vi "Not A Refnum.vi"(8 "error in (no error)":errorcluster, 11 "Log File in":refnum<class "Log File.lvclass">) -> (0 "error out":errorcluster, 2 "Not a Refnum?":bool, 3 "Log File out":refnum<class "Log File.lvclass">)   [LabVIEW 2015, in "Log File.lvclass"]
uses:
  Log File.lvclass
  Log File.lvclass/Log File.ctl
  TDMS Log File/TDMS Log File.lvclass
  Text Log File/Text Log File.lvclass
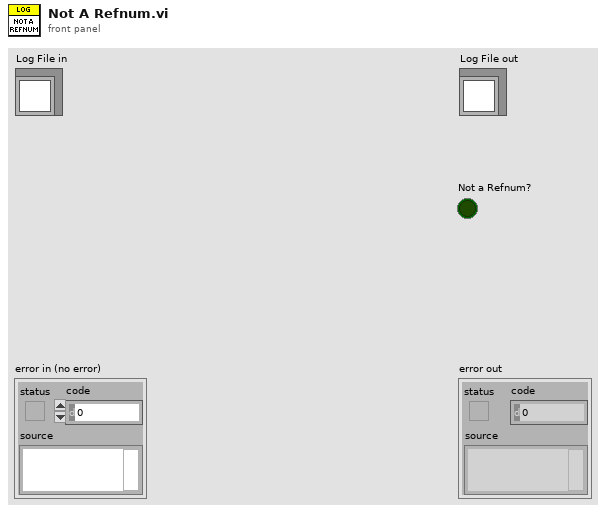
[diagram p1: front panel]
types:
  T1 = typedef "Log File.lvclass/Log File Type.ctl" = enum16{"Default", "TDMS", "Text"}
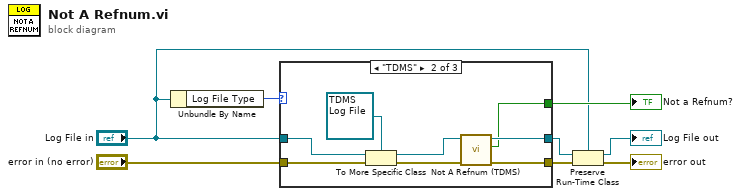
[diagram p0: block diagram]
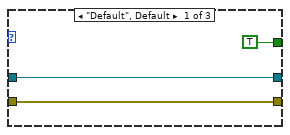
[diagram p2: hidden frame]
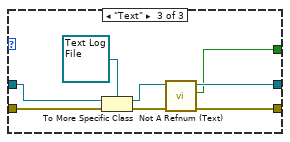
[diagram p3: hidden frame]
diagram:
  n1 = Unbundle By Name("Log File in") -> ("Log File Type"=w8:T1)
  n2 = case shown="\"TDMS\"" w8 {
    tunnel: "error in (no error)" -> [w11 w19 w26]
    tunnel: [w11 w14 w27] -> w5
    tunnel: "Log File in" -> [w10 w18 w24]
    tunnel: [w10 w13 w21] -> w4
    tunnel: [TRUE ("Not a Refnum?") w12 w20] -> w6
    frame "Default", Default {
    }
    frame "TDMS" {
      n3 = To More Specific Class(target class=refnum<class "TDMS Log File.lvclass"> refnum ("TDMS Log File.lvclass"), reference=w18, error in=w19) -> (specific class reference=w16:refnum<class "TDMS Log File.lvclass">, error out=w15:errorcluster)
      n4 = call "Not A Refnum (TDMS).vi"("error in (no error)"=w15, "TDMS Log File in"=w16) -> ("error out"=w14:errorcluster, "Not a Refnum?"=w12:bool, "TDMS Log File out"=w13:refnum<class "TDMS Log File.lvclass">)  [unwired: 7 in]
    }
    frame "Text" {
      n5 = To More Specific Class(target class=refnum<class "Text Log File.lvclass"> refnum ("Text Log File.lvclass"), reference=w24, error in=w26) -> (specific class reference=w22:refnum<class "Text Log File.lvclass">, error out=w25:errorcluster)
      n6 = call "Not A Refnum (Text).vi"("error in (no error)"=w25, "Text Log File in"=w22) -> ("error out"=w27:errorcluster, "Not a Refnum?"=w20:bool, "Text Log File out"=w21:refnum<class "Text Log File.lvclass">)  [unwired: 7 in]
    }
  }
  "Not a Refnum?" <- w6
  n7 = Preserve Run-Time Class(object in=w4, error in=w5, 2:"Log File in") -> (object out=→"Log File out":refnum<class "Log File.lvclass">, error out=→"error out":errorcluster)
